vi "MSB LSB.vi"(10 "Array in":u8[](array[numeric]), 11 "Hex Array Out":string[](array[string])) -> (3 "Array out":u16[](array[numeric]))   [LabVIEW 2016]
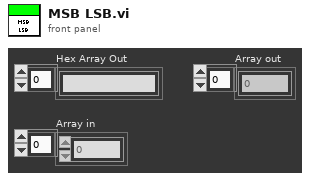
[diagram p1: front panel]
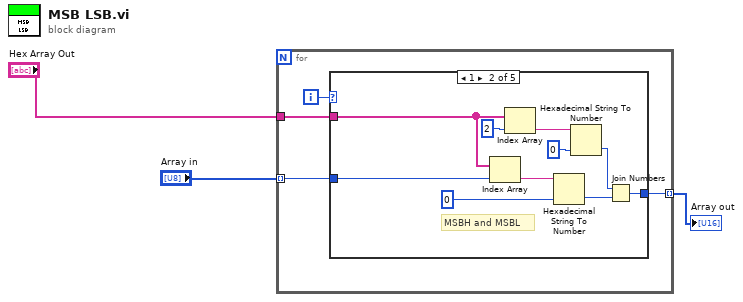
[diagram p0: block diagram]
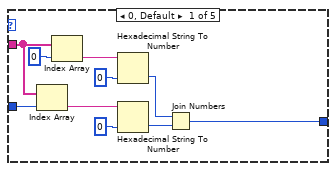
[diagram p2: hidden frame]
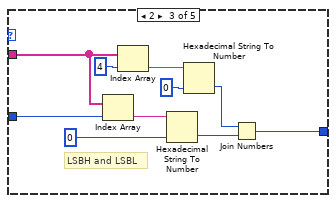
[diagram p3: hidden frame]
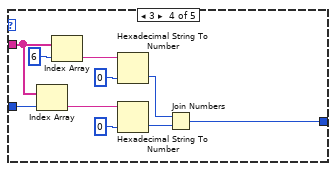
[diagram p4: hidden frame]
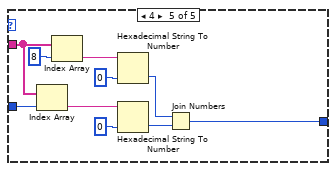
[diagram p5: hidden frame]
diagram:
  n1 = for {
    tunnel: "Hex Array Out" -> [w7]
    tunnel: "Array in" -> [w6] mode=indexing
    tunnel: [w4] -> w3 mode=indexing
    i -> [w5]
    n2 = case shown="1" w5 {
      tunnel: w7 -> [w12 w23 w30 w40 w50]
      tunnel: w6 -> [w11 w22 w29 w38 w49]
      tunnel: [w15 w18 w28 w39 w48] -> w4
      frame 0, Default {
        n3 = Index Array(array=w12, index=w11) -> (element=w10:string)
        n4 = Index Array(array=w12, index=0) -> (element=w14:string)
        n5 = Hexadecimal String To Number(string=w14, default (0uL)=u8 0 ("default (0 U32)")) -> (number=w17:u8)  [unwired: 1 in, 1 out]
        n6 = Hexadecimal String To Number(string=w10, default (0uL)=u8 0 ("default (0 U32)")) -> (number=w8:u8)  [unwired: 1 in, 1 out]
        n7 = Join Numbers(hi=w17, lo=w8) -> ((hi.lo)=w15:u16)
      }
      frame 1 {
        # "MSBH and MSBL"
        n8 = Index Array(array=w23, index=w22) -> (element=w21:string)
        n9 = Index Array(array=w23, index=2) -> (element=w24:string)
        n10 = Hexadecimal String To Number(string=w21, default (0uL)=u8 0 ("default (0 U32)")) -> (number=w19:u8)  [unwired: 1 in, 1 out]
        n11 = Hexadecimal String To Number(string=w24, default (0uL)=u8 0 ("default (0 U32)")) -> (number=w27:u8)  [unwired: 1 in, 1 out]
        n12 = Join Numbers(hi=w27, lo=w19) -> ((hi.lo)=w18:u16)
      }
      frame 2 {
        # "LSBH and LSBL"
        n13 = Index Array(array=w30, index=w29) -> (element=w33:string)
        n14 = Index Array(array=w30, index=4) -> (element=w34:string)
        n15 = Hexadecimal String To Number(string=w33, default (0uL)=u8 0 ("default (0 U32)")) -> (number=w31:u8)  [unwired: 1 in, 1 out]
        n16 = Hexadecimal String To Number(string=w34, default (0uL)=u8 0 ("default (0 U32)")) -> (number=w37:u8)  [unwired: 1 in, 1 out]
        n17 = Join Numbers(hi=w37, lo=w31) -> ((hi.lo)=w28:u16)
      }
      frame 3 {
        n18 = Index Array(array=w40, index=w38) -> (element=w43:string)
        n19 = Index Array(array=w40, index=6) -> (element=w44:string)
        n20 = Hexadecimal String To Number(string=w44, default (0uL)=u8 0 ("default (0 U32)")) -> (number=w47:u8)  [unwired: 1 in, 1 out]
        n21 = Hexadecimal String To Number(string=w43, default (0uL)=u8 0 ("default (0 U32)")) -> (number=w41:u8)  [unwired: 1 in, 1 out]
        n22 = Join Numbers(hi=w47, lo=w41) -> ((hi.lo)=w39:u16)
      }
      frame 4 {
        n23 = Index Array(array=w50, index=w49) -> (element=w53:string)
        n24 = Index Array(array=w50, index=8) -> (element=w54:string)
        n25 = Hexadecimal String To Number(string=w54, default (0uL)=u8 0 ("default (0 U32)")) -> (number=w57:u8)  [unwired: 1 in, 1 out]
        n26 = Hexadecimal String To Number(string=w53, default (0uL)=u8 0 ("default (0 U32)")) -> (number=w51:u8)  [unwired: 1 in, 1 out]
        n27 = Join Numbers(hi=w57, lo=w51) -> ((hi.lo)=w48:u16)
      }
    }
  }
  "Array out" <- w3
